vi "temp.vi"(7 "error in":errorcluster) -> (27 "error out":errorcluster)   [LabVIEW 2018]
uses:
  <vilib>/vision/Pattern Matching.llb/IMAQ Pattern Match Advanced Options.ctl
  <vilib>/vision/NI_Vision_Development_Module.lvlib
panel:
  out "Image Out":T1(plugin-control)
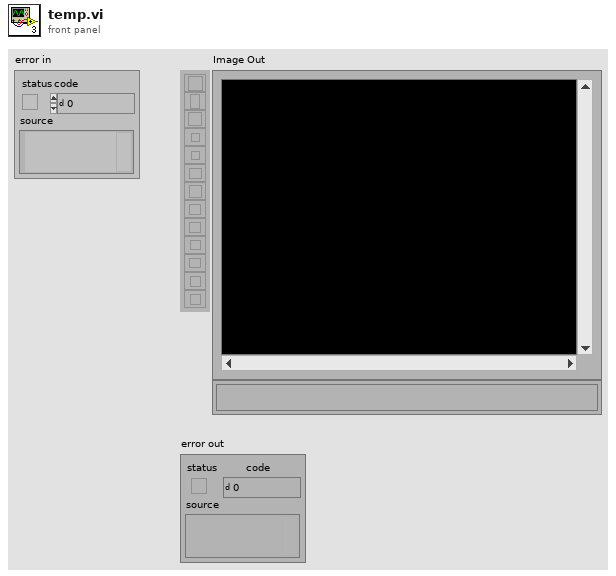
[diagram p1: front panel]
types:
  T1 = typedef "IMAQ Image.ctl" = refnum<image>
  T2 = cluster{"Feature":u32, "Points IDs":cluster{"GUID":string, "Index":i32}[]}[]
  T3 = enum16{"Get First Edge", "Get First + Last Edge", "Get All Edges"}
  T4 = cluster{"Level Type":enum32{"Absolute Value", "Relative value"}, "Threshold Level":i32, "Hysteresis":i32}
  T5 = cluster{"Global Rectangle":i32[], "Contours":cluster{"ID":enum32{"External", "Internal"}, "Type":u32, "Coordinates":i32[]}[]}
  T6 = typedef "IMAQ Pattern Match Advanced Options.ctl" = u16
  T7 = cluster{"Number of Matches Requested":i32, "Minimum Match Score":sgl, "Angle Ranges":cluster{"Start Angle":sgl, "End Angle":sgl}[]}
  T8 = typedef "Image Type" = u32
  T9 = cluster{"Position":cluster{"x":sgl, "y":sgl}, "Angle":sgl, "Scale":sgl, "Score":sgl, "Bounding Box":cluster{"x":sgl, "y":sgl}[]}[]
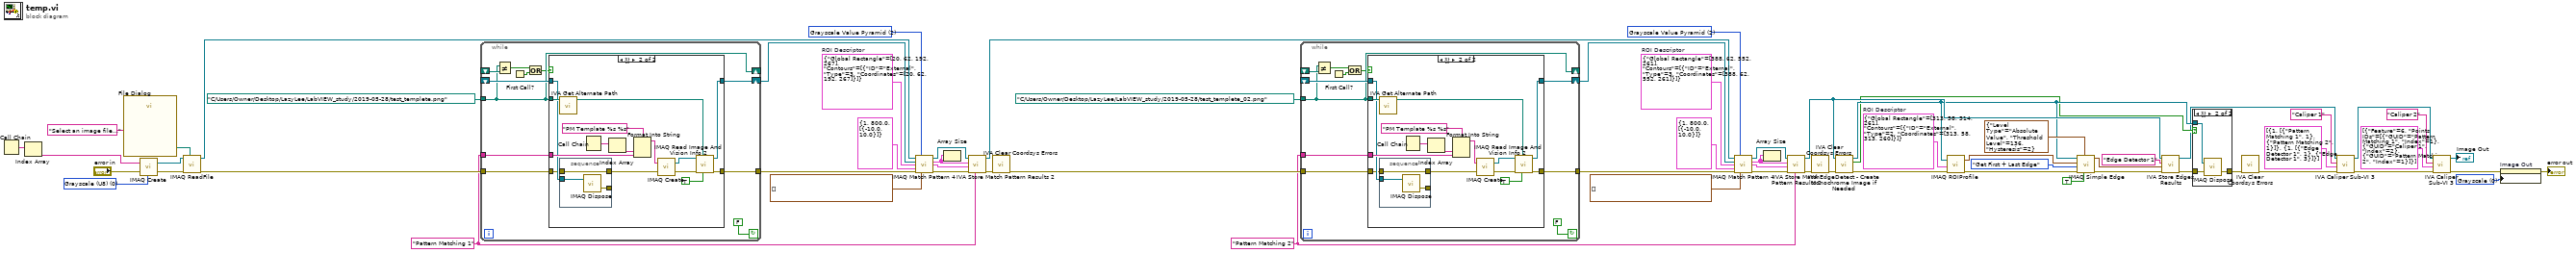
[diagram p0: block diagram]
diagram:
  w1 = u32 0 items=["Grayscale", "Binary", "Gradient", "Rainbow", "Temperature", "User Defined", "Binary 16 Bit", "Gradient 16 Bit", "Rainbow 16 Bit", "Temperature 16 Bit", "User Defined 16 Bit"] ("Palette Type")
  w22 = T5 {"Global Rectangle"=[313, 58, 314, 261], "Contours"=[{"ID"=enum."External", "Type"=2, "Coordinates"=[313, 58, 313, 260]}]}  # ROI Descriptor
  w38 = 2 items=["All", "Low Discrepancy Sampling", "Grayscale Value Pyramid", "Gradients Pyramid"] ("Algorithm")
  w35 = "Pattern Matching 2" ("Step Name")
  w37 = T5 {"Global Rectangle"=[388, 62, 552, 261], "Contours"=[{"ID"=enum."External", "Type"=3, "Coordinates"=[388, 62, 552, 261]}]}  # ROI Descriptor
  w53 = 2 items=["All", "Low Discrepancy Sampling", "Grayscale Value Pyramid", "Gradients Pyramid"] ("Algorithm")
  w50 = "Pattern Matching 1" ("Step Name")
  w52 = T5 {"Global Rectangle"=[20, 62, 192, 267], "Contours"=[{"ID"=enum."External", "Type"=3, "Coordinates"=[20, 62, 192, 267]}]}  # ROI Descriptor
  w58 = T8 0 items=["Grayscale (U8)", "Grayscale (I16)", "Grayscale (SGL)", "Complex (CSG)", "RGB (U32)", "HSL (U32)", "RGB (U64)", "Grayscale (U16)"] ("Image Type")
  n1 = Call Chain() -> (call chain=w62:string[])
  n2 = Index Array(array=w62) -> (element=w61:string)  [unwired: 1 in]
  n3 = call "File Dialog"("prompt"="Select an image file...") -> ("selected path"=w59:path)  [unwired: 6 in, 8 out]
  n4 = call "IMAQ Create"("Image Name"=w61, "Image Type"=w58, "error in (no error)"="error in") -> ("New Image"=w65:T1, "error out"=w64:errorcluster)  [unwired: 1 in, 1 out]
  n5 = call "IMAQ ReadFile"("File Path"=w59, "error in (no error)"=w64, "Image"=w65) -> ("error out"=w66:errorcluster, "Image Out"=w56:T1)  [unwired: 2 in, 5 out]
  n6 = while {
    shift-right: [w77] -> w47
    shift-left: _ -> [w76]
    tunnel: [w74] -> w46
    tunnel: w66 -> [w73]
    tunnel: path "C:/Users/Owner/Desktop/LazyLee/LabVIEW_study/2019-05-28/test_templete.png" ("Template File Path") -> [w70]
    tunnel: w50 -> [w72]
    shift-right: [w70] -> _
    shift-left: _ -> [w71]
    stop <- FALSE continue-if-true
    n7 = Not Equal?(x=w70, y=w71) -> (x != y?=w68:bool)
    n8 = First Call?() -> (First Call?: T/F=w69:bool)
    n9 = Or(x=w68, y=w69) -> (x .or. y?=w67:bool)
    n10 = case "케이스 구조" shown="참" w67 {
      tunnel: [w79 w84] -> w77
      tunnel: w76 -> [w79 w88]
      tunnel: [w78 w85] -> w74
      tunnel: w73 -> [w78 w87]
      tunnel: w70 -> [_ w89]
      tunnel: w72 -> [_ w90]
      frame False {
      }
      frame True {
        n11 = call <vilib>:"IVA Get Alternate Path.vi"("Path In"=w89) -> ("Path Out"=w86:path)  [unwired: 10 out]
        n12 = stacked-sequence "다층 시퀀스 구조" {
          tunnel: w88 -> [w97]
          tunnel: w87 -> [w96]
          tunnel: [w96] -> w81
          tunnel: [w95] -> _
          frame #0 {
            n13 = call "IMAQ Dispose"("Image"=w97) -> ("error out"=w95:errorcluster)  [unwired: 2 in, 3 out]
          }
        }
        n14 = Call Chain() -> (call chain=w92:string[])
        n15 = Index Array(array=w92) -> (element=w91:string)  [unwired: 1 in]
        n16 = Format Into String(format string="PM Template %s %s" ("Image Name"), w91, w90) -> (resulting string=w94:string)  [unwired: 2 in, 1 out]
        n17 = call "IMAQ Create"("Image Name"=w94, "error in (no error)"=w81) -> ("New Image"=w83:T1, "error out"=w82:errorcluster)  [unwired: 2 in, 1 out]
        n18 = call "IMAQ Read Image And Vision Info 2"("Use File Path Image Type"=TRUE, "File Path"=w86, "error in (no error)"=w82, "Image"=w83) -> ("error out"=w85:errorcluster, "Image Out"=w84:T1)  [unwired: 5 in, 1 out]
      }
    }
  }
  n19 = call "IMAQ Match Pattern 4"("Image"=w56, "Algorithm"=w53, "Template Image"=w47, "ROI Descriptor"=w52, "Parameters"=T7 {"Number of Matches Requested"=1, "Minimum Match Score"=800.0, "Angle Ranges"=[{"Start Angle"=-10.0, "End Angle"=10.0}]}, "error in (no error)"=w46, "Advanced Options"=cluster{"Item":T6, "Value":dbl}[] []) -> ("Image (duplicate)"=w54:T1, "Matches (pixel)"=w49:T9, "Matches (real-world)"=w48:T9, "error out"=w55:errorcluster)  [unwired: 4 in, 1 out]
  n20 = Array Size(array=w49) -> ()  [unwired: 1 out]
  n21 = call <vilib>:"IVA Store Match Pattern Results 2.vi"("Step Name"=w50, "error in (no error)"=w55, "Matches (real-world)"=w48, "Matches (pixel)"=w49, "Image in"=w54) -> ("error out"=w45:errorcluster, "Image dup"=w41:T1)  [unwired: 1 in, 4 out]
  n22 = call <vilib>:"IVA Clear Coordsys Errors.vi"("error in (no error)"=w45) -> ("error out"=w44:errorcluster)  [unwired: 10 in]
  n23 = while {
    shift-right: [w108] -> w32
    shift-left: _ -> [w107]
    tunnel: [w105] -> w31
    tunnel: w44 -> [w104]
    tunnel: path "C:/Users/Owner/Desktop/LazyLee/LabVIEW_study/2019-05-28/test_templete_02.png" ("Template File Path") -> [w101]
    tunnel: w35 -> [w103]
    shift-right: [w101] -> _
    shift-left: _ -> [w102]
    stop <- FALSE continue-if-true
    n24 = Not Equal?(x=w101, y=w102) -> (x != y?=w99:bool)
    n25 = First Call?() -> (First Call?: T/F=w100:bool)
    n26 = Or(x=w99, y=w100) -> (x .or. y?=w98:bool)
    n27 = case "케이스 구조" shown="참" w98 {
      tunnel: [w110 w115] -> w108
      tunnel: w107 -> [w110 w119]
      tunnel: [w109 w116] -> w105
      tunnel: w104 -> [w109 w118]
      tunnel: w101 -> [_ w120]
      tunnel: w103 -> [_ w121]
      frame False {
      }
      frame True {
        n28 = call <vilib>:"IVA Get Alternate Path.vi"("Path In"=w120) -> ("Path Out"=w117:path)  [unwired: 10 out]
        n29 = stacked-sequence "다층 시퀀스 구조" {
          tunnel: w119 -> [w128]
          tunnel: w118 -> [w127]
          tunnel: [w127] -> w112
          tunnel: [w126] -> _
          frame #0 {
            n30 = call "IMAQ Dispose"("Image"=w128) -> ("error out"=w126:errorcluster)  [unwired: 2 in, 3 out]
          }
        }
        n31 = Call Chain() -> (call chain=w123:string[])
        n32 = Index Array(array=w123) -> (element=w122:string)  [unwired: 1 in]
        n33 = Format Into String(format string="PM Template %s %s" ("Image Name"), w122, w121) -> (resulting string=w125:string)  [unwired: 2 in, 1 out]
        n34 = call "IMAQ Create"("Image Name"=w125, "error in (no error)"=w112) -> ("New Image"=w114:T1, "error out"=w113:errorcluster)  [unwired: 2 in, 1 out]
        n35 = call "IMAQ Read Image And Vision Info 2"("Use File Path Image Type"=TRUE, "File Path"=w117, "error in (no error)"=w113, "Image"=w114) -> ("error out"=w116:errorcluster, "Image Out"=w115:T1)  [unwired: 5 in, 1 out]
      }
    }
  }
  n36 = call "IMAQ Match Pattern 4"("Image"=w41, "Algorithm"=w38, "Template Image"=w32, "ROI Descriptor"=w37, "Parameters"=T7 {"Number of Matches Requested"=1, "Minimum Match Score"=800.0, "Angle Ranges"=[{"Start Angle"=-10.0, "End Angle"=10.0}]}, "error in (no error)"=w31, "Advanced Options"=cluster{"Item":T6, "Value":dbl}[] []) -> ("Image (duplicate)"=w39:T1, "Matches (pixel)"=w34:T9, "Matches (real-world)"=w33:T9, "error out"=w40:errorcluster)  [unwired: 4 in, 1 out]
  n37 = Array Size(array=w34) -> ()  [unwired: 1 out]
  n38 = call <vilib>:"IVA Store Match Pattern Results 2.vi"("Step Name"=w35, "error in (no error)"=w40, "Matches (real-world)"=w33, "Matches (pixel)"=w34, "Image in"=w39) -> ("error out"=w30:errorcluster, "Image dup"=w20:T1)  [unwired: 1 in, 4 out]
  n39 = call <vilib>:"IVA Clear Coordsys Errors.vi"("error in (no error)"=w30) -> ("error out"=w29:errorcluster)  [unwired: 10 in]
  n40 = call <vilib>:"IVA EdgeDetect - Create Monochrome Image if Needed.vi"("error in (no error)"=w29, "Image In"=w20) -> ("error out"=w16:errorcluster, "Mono Image Created"=w14:bool, "Mono Image Out"=w15:T1)  [unwired: 7 out]
  n41 = call "IMAQ ROIProfile"("error in (no error)"=w16, "ROI Descriptor"=w22, "Image"=w15) -> ("error out"=w17:errorcluster, "Pixel Coordinates"=w18:cluster{"X":u32, "Y":u32}[])  [unwired: 4 out]
  n42 = call "IMAQ Simple Edge"("Sub-Pixel Accuracy"=TRUE, "Threshold Parameters"=T4 {"Level Type"=enum."Absolute Value", "Threshold Level"=136, "Hysteresis"=2}, "error in (no error)"=w17, "Process"=T3."Get First + Last Edge", "Pixel Coordinates"=w18, "Image Src"=w15) -> ("error out"=w23:errorcluster, "Edges Coordinates"=w24:cluster{"X":sgl, "Y":sgl}[])  [unwired: 4 out]
  n43 = call <vilib>:"IVA Store Edges Results.vi"("error in (no error)"=w23, "Edge Coordinates"=w24, "Step Name"="Edge Detector 1", "Image in"=w20) -> ("error out"=w13:errorcluster, "Image dup"=w11:T1)  [unwired: 6 out]
  n44 = case "케이스 구조" shown="참" w14 {
    tunnel: w15 -> [_ w132]
    tunnel: w13 -> [w129 w131]
    tunnel: [w129 w130] -> w12
    frame False {
    }
    frame True {
      n45 = call "IMAQ Dispose"("Image"=w132, "error in (no error)"=w131) -> ("error out"=w130:errorcluster)  [unwired: 1 in, 3 out]
    }
  }
  n46 = call <vilib>:"IVA Clear Coordsys Errors.vi"("error in (no error)"=w12) -> ("error out"=w19:errorcluster)  [unwired: 10 in]
  n47 = call <vilib>:"IVA Caliper Sub-VI 3.vi"("error in"=w19, "Parameters"=T2 [{"Feature"=1, "Points IDs"=[{"GUID"="Pattern Matching 1", "Index"=1}, {"GUID"="Pattern Matching 2", "Index"=1}]}, {"Feature"=1, "Points IDs"=[{"GUID"="Edge Detector 1", "Index"=1}, {"GUID"="Edge Detector 1", "Index"=3}]}], "Step Name"="Caliper 1", "Image In"=w11) -> ("error out"=w10:errorcluster, "Image Out"=w7:T1)  [unwired: 1 in, 5 out]
  n48 = call <vilib>:"IVA Caliper Sub-VI 3.vi"("error in"=w10, "Parameters"=T2 [{"Feature"=6, "Points IDs"=[{"GUID"="Pattern Matching 1", "Index"=1}, {"GUID"="Caliper 1", "Index"=2}, {"GUID"="Pattern Matching 2", "Index"=1}]}], "Step Name"="Caliper 2", "Image In"=w7) -> ("error out"=w6:errorcluster, "Image Out"=→"Image Out":T1)  [unwired: 1 in, 5 out]
  n49 = property on="Image Out" class="ImageControl"(error in=w6, "Palette:Palette Type"=w1) -> (error out=→"error out":errorcluster)  [unwired: 1 in, 1 out]
